vi "HeaderFluorescence.vi"(9 "N APD Samp/step":i32=3, 10 "APD Integration Time (s)":dbl=0.01 caption="Integration Time (s)", 11 "Trap Path":path) -> (3 "Flu File":refnum<file>)   [LabVIEW 2013]
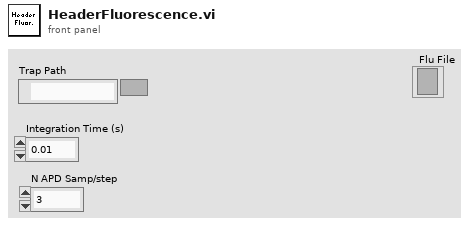
[diagram p1: front panel]
types:
  T1 = enum16{"big-endian, network order", "native, host order", "little-endian"}
  T2 = enum16{"open", "replace", "create", "open or create", "replace or create", "replace or create with confirmation"}
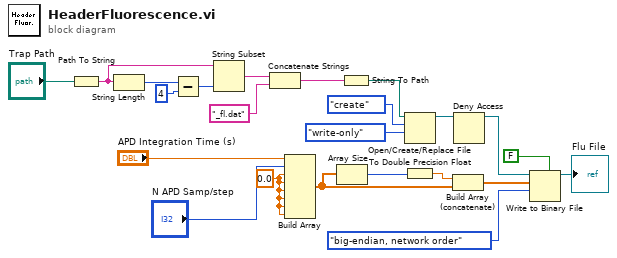
[diagram p0: block diagram]
diagram:
  w1 = 0.0
  n1 = Path To String(path="Trap Path") -> (string=w5:string)
  n2 = String Length(string=w5) -> (length=w6:i32)
  n3 = Subtract(x=w6, y=4) -> (x-y=w8:i32)
  n4 = String Subset(string=w5, length (rest)=w8) -> (substring=w9:string)  [unwired: 1 out]
  n5 = Concatenate Strings(w9, "_fl.dat" ("string")) -> (w11:string)
  n6 = Build Array("APD Integration Time (s)", "N APD Samp/step", w1, w1, w1, w1, w1, w1) -> (w21:dbl[])
  n7 = Array Size(array=w21) -> (size(s)=w19:i32)
  n8 = String To Path(string=w11) -> (path=w15:path)
  n9 = Open/Create/Replace File(file path (use dialog)=w15, operation (0:open)=T2."create", access (0:read/write)=enum16{"read/write", "read-only", "write-only"}."write-only") -> (refnum out=w14:refnum<file>)  [unwired: 1 in, 4 out]
  n10 = To Double Precision Float(number=w19) -> (double precision float=w20:dbl)
  n11 = Build Array (concatenate)(w20, w21) -> (w22:dbl[])
  n12 = Deny Access(7:w14) -> (3:w18:refnum<file>)  [unwired: 1 in, 2 out]
  n13 = Write to Binary File(file (use dialog)=w18, data=w22, 5:FALSE ("prepend array or string size? (T)"), 9:T1."big-endian, network order" ("byte order (0:big-endian, network order)")) -> (refnum out=→"Flu File":refnum<file>)  [unwired: 1 in, 3 out]
